vi "Align Decide.vi"() -> (3 "Next Step":T1)   [LabVIEW 2014]
uses:
  Common Code/Inner Roller States.ctl
  Common Code/Change Detect Int.vi
  Robot Global Data.vi
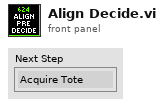
[diagram p1: front panel]
types:
  T1 = typedef "Inner Roller States.ctl" = enum16{"Acquire Tote", "Absorb Tote", "Turn Tote Right", "Turn Tote Left"}
  T2 = typedef "Dashboard Control Data.ctl" = cluster{"Cam Exposure":dbl, "Go to angle":dbl, "Steer PID Gains":cluster{"proportional gain (Kc)":dbl, "integral time (Ti, min)":dbl, "derivative time (Td, min)":dbl}, "Steer PID output Range":cluster{"output high":dbl, "output low":dbl}, "Pressure m \nValue":dbl, "Pressure b \nValue":dbl, "Roller Command Cluster ":T3, "Elevator":T4, "Encoder Control":T6, "IMU Controls":cluster{"Pitch Zero":dbl, "Roll Zero":dbl}, "Auton Settings":cluster{"Drive Dist Window Size":dbl}, "Drivetrain Settings":T7}
  T3 = typedef "Roller Control.ctl" = cluster{"Intake Speed":dbl, "Turn In Speed":dbl, "Unload Speed":dbl, "Turn Out Speed":dbl, "Ping Align Tolerance":dbl, "Tote Range Threshold":dbl, "Right Pot 0":dbl, "Pot Threshold":dbl, "Left Pot 0":dbl, "Manual 0s?":bool, "Right Pot Scale":dbl, "Left Pot Scale":dbl, "0 wait time":i32, "Zero Pots":bool, "Min Elevator Height":dbl, "Eject Time":dbl, "Eject US Threshold":dbl, "Anti-Twitch Time":u32, "Ping Caring Threshold":dbl, "Pot Diff Threshold":dbl, "Pinch Sustain":u32, "Absorb Give Up Threshold":dbl, "Untip In Threshold":dbl, "Untip Grab Range":dbl}
  T4 = typedef "Elevator DB Control.ctl" = cluster{"PID Output Range":cluster{"output high":dbl, "output low":dbl}, "PID gains":cluster{"proportional gain (Kc)":dbl, "integral time (Ti, min)":dbl, "derivative time (Td, min)":dbl}, "Height Tolerance":sgl, " Encoder Constant":dbl, "Safe Mode Max Speed":sgl, "Eject Time":sgl, "Zeroing Speed":sgl, "Presets":T5, "Ping Detect Threshold":sgl, "Trashcan Detect Threshold":sgl, "Zero Filter Time":dbl, "Stabilizer Open Time":dbl}
  T5 = typedef "Elevator Presets.ctl" = cluster{"Hold Tote":sgl, "Hold Trashcan":sgl, "Pickup 2 w/ Tote":sgl, "Pickup 2 w/ Trashcan":sgl, "Pickup 3 w/ Tote":sgl, "Pickup 3 w/ Trashcan":sgl, "Bottom":sgl, "Pickup 1 w/ Tote":sgl, "Pickup Trashcan":sgl, "Pickup 1 w/ Trashcan":sgl, "Eject":sgl, "Hold Low":sgl, "Step add height":sgl, "Store Trashcan 3":sgl, "Store Trashcan 4":sgl, "Store Trashcan 5":sgl, "6 Tote Max Height":sgl, "5 Tote Max Height":sgl, "Idle Empty":dbl, "Untip Lift":dbl, "Drop Stack":dbl}
  T6 = typedef "Encoder Control.ctl" = cluster{"Left Tick Constant":dbl, "Right Tick Constant":dbl, "Center Tick Constant":dbl, "Reset?":bool, "Y Dist":cluster{"PID gains":cluster{"proportional gain (Kc)":dbl, "integral time (Ti, min)":dbl, "derivative time (Td, min)":dbl}, "output range":cluster{"output high":dbl, "output low":dbl}}, "X Dist":cluster{"PID gains":cluster{"proportional gain (Kc)":dbl, "integral time (Ti, min)":dbl, "derivative time (Td, min)":dbl}, "output range":cluster{"output high":dbl, "output low":dbl}}, "Y Stop Thresh":dbl, "Y Stop Speed":dbl, "X Stop Thresh":dbl, "X Stop Speed":dbl}
  T7 = typedef "Drivetrain Settings.ctl" = cluster{"Gyro Tolerance":dbl, "Strafe Correct max steer":dbl, "Strafe Timer Wait":dbl, "Throttle Ramp (ms)":dbl, "Strafe Ramp (ms)":dbl}
  T8 = typedef "Ultrasonic Indicators.ctl" = cluster{"Left Distance":dbl, "Right Distance":dbl, "Center Distance":dbl}
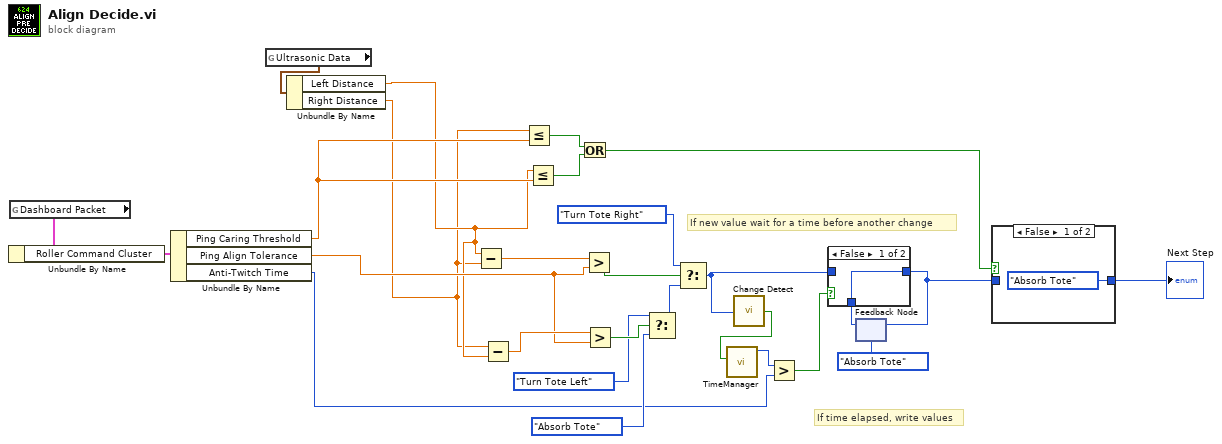
[diagram p0: block diagram]
diagram:
  # "If time elapsed, write values"
  # "If new value wait for a time before another change"
  n1 = global read "Robot Global Data.vi" "Dashboard Packet"() -> (w19:T2)
  n2 = Unbundle By Name(w19) -> ("Roller Command Cluster"=w18:T3)
  n3 = Unbundle By Name(w18) -> ("Ping Caring Threshold"=w7:dbl, "Ping Align Tolerance"=w17:dbl, "Anti-Twitch Time"=w15:u32)
  n4 = global read "Robot Global Data.vi" "Ultrasonic Data"() -> (w3:T8)
  n5 = Unbundle By Name(w3) -> ("Left Distance"=w2:dbl, "Right Distance"=w1:dbl)
  n6 = Subtract(x=w2, y=w1) -> (x-y=w27:dbl)
  n7 = Subtract(x=w1, y=w2) -> (x-y=w26:dbl)
  n8 = Less Or Equal?(x=w1, y=w7) -> (x <= y?=w9:bool)
  n9 = Less Or Equal?(x=w2, y=w7) -> (x <= y?=w8:bool)
  n10 = Or(x=w9, y=w8) -> (x .or. y?=w6:bool)
  n11 = Greater?(x=w27, y=w17) -> (0:w24:bool)
  n12 = Greater?(x=w26, y=w17) -> (0:w23:bool)
  n13 = Select(t=Inner_Roller_States."Turn Tote Left", s=w23, f=Inner_Roller_States."Absorb Tote") -> (s? t:f=w25:T1)
  n14 = Select(t=Inner_Roller_States."Turn Tote Right", s=w24, f=w25) -> (s? t:f=w12:T1)
  n15 = call-poly "Change Detect.vi"("In"=w12) -> ("Changed?"=w14:bool)
  n16 = call "TimeManager.vi"("Reset?"=w14) -> ("Time Since Reset"=w16:u32)  [unwired: 9 in, 1 out]
  n17 = Greater?(x=w16, y=w15) -> (0:w13:bool)
  n18 = feedback #1(Inner_Roller_States."Absorb Tote") -> (w11:T1)
  n19 = case shown="False" w13 {
    tunnel: w12 -> [_ w29]
    tunnel: [w28 w29] -> w4
    tunnel: w11 -> [w28 _]
    frame False {
    }
    frame True {
    }
  }
  n20 = feedback-in #1(w4) -> ()
  n21 = case shown="False" w6 {
    tunnel: [Inner_Roller_States."Absorb Tote" w31] -> w5
    tunnel: w4 -> [_ w31]
    frame False {
    }
    frame True {
    }
  }
  "Next Step" <- w5
